vi "step3N.vi"(1 "NT":u32, 2 "C1":bool, 3 "NC1":u32, 4 "C2":bool, 5 "NC2":u32, 6 "T":u32, 7 "C3":bool, 8 "T NT2":u32[][](array[numeric])=[[0, 0]], 9 "NC3":u32, 10 "C NC2":cluster{"C":bool, "NC":u32}[][](array[cluster])=[[{"C"=FALSE, "NC"=0}, {"C"=FALSE, "NC"=0}, {"C"=FALSE, "NC"=0}]], 12 "N step":u32) -> (14 "T NT":u32[][](array[numeric]), 15 "C NC":cluster{"C":bool, "NC":u32}[][](array[cluster]))   [LabVIEW 2019, in "Userlib.lvlib"]
uses:
  Userlib.lvlib
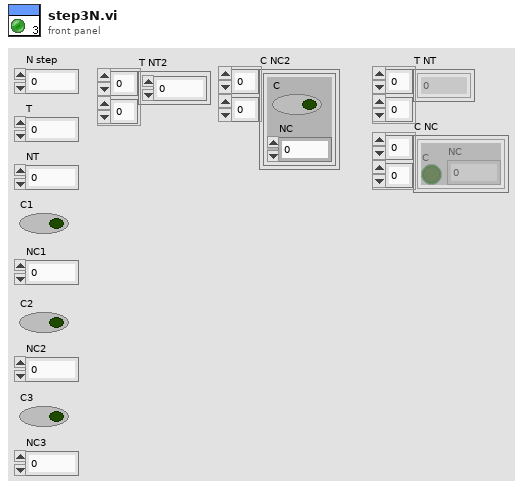
[diagram p1: front panel]
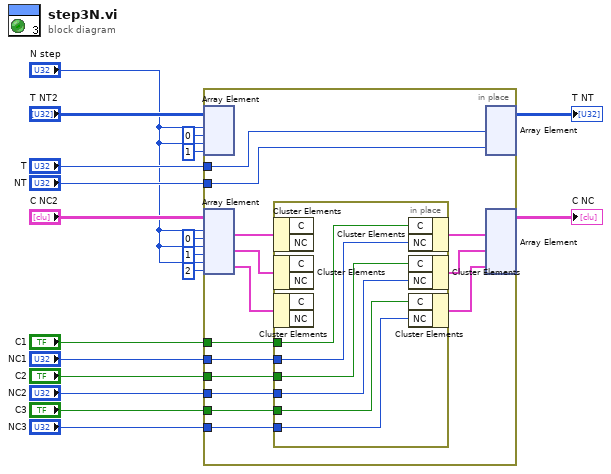
[diagram p0: block diagram]
diagram:
  n1 = in-place {
    in-place-border: "T" -> [w32]
    in-place-border: "NT" -> [w31]
    in-place-border: "C1" -> [w24]
    in-place-border: "NC1" -> [w23]
    in-place-border: "C2" -> [w22]
    in-place-border: "NC2" -> [w21]
    in-place-border: "C3" -> [w20]
    in-place-border: "NC3" -> [w19]
    n2 = in-place-array #1("T NT2", "N step", 0, "N step", 1) -> ()  [unwired: 2 out]
    n3 = in-place-array #2("C NC2", "N step", 0, "N step", 1, "N step", 2) -> (w30:cluster{"C":bool, "NC":u32}, w29:cluster{"C":bool, "NC":u32}, w28:cluster{"C":bool, "NC":u32})
    n4 = in-place {
      in-place-border: w24 -> [w38]
      in-place-border: w23 -> [w37]
      in-place-border: w22 -> [w36]
      in-place-border: w21 -> [w35]
      in-place-border: w20 -> [w34]
      in-place-border: w19 -> [w33]
      n5 = in-place-cluster #3(w30) -> ()  [unwired: 2 out]
      n6 = in-place-cluster #4(w29) -> ()  [unwired: 2 out]
      n7 = in-place-cluster #5(w28) -> ()  [unwired: 2 out]
      n8 = in-place-cluster #3("C"=w38, "NC"=w37) -> (w27:cluster{"C":bool, "NC":u32})
      n9 = in-place-cluster #4("C"=w36, "NC"=w35) -> (w26:cluster{"C":bool, "NC":u32})
      n10 = in-place-cluster #5("C"=w34, "NC"=w33) -> (w25:cluster{"C":bool, "NC":u32})
    }
    n11 = in-place-array #1(w32, w31) -> (→"T NT":u32[][])  [unwired: 4 out]
    n12 = in-place-array #2(w27, w26, w25) -> (→"C NC":cluster{"C":bool, "NC":u32}[][])  [unwired: 6 out]
  }
